vi "finlfinal1`.vi"() -> ()   [LabVIEW 2020]
uses:
  <vilib>/DAQmx/read.llb/DAQmx Read (Digital Bool 1Line 1Point).vi
  <vilib>/DAQmx/read.llb/DAQmx Read (Analog DBL 1Chan 1Samp).vi
  <vilib>/DAQmx/create/channels.llb/DAQmx Create Channel (AI-Voltage-Basic).vi
  <vilib>/DAQmx/create/channels.llb/DAQmx Create Channel (DI-Digital Input).vi
  <vilib>/Instr/_visa.llb/VISA Configure Serial Port (Instr).vi
  <vilib>/DAQmx/miscellaneous.llb/DAQmx Fill In Error Info.vi
  <vilib>/httpClient/PUTBuffer.vi
  <vilib>/httpClient/LabVIEWHTTPClient.lvlib
panel:
  in  "VISA resource name":refnum<visa-resource-name>
  in  "Bottle Presence":tag
  in  "Temperature":tag
  out "Temperature":dbl
  out "Humidity":dbl
  out "Temperature":dbl(knob) caption="Meter" scale=0.0..150.0
  out "Humidity Chart":dbl(graph)
  in  "Dispense Trigger":bool
  in  "Dispensing":bool
  out "error out":errorcluster
  out "Ready to Dispense":bool
  out "Temp Safe":bool
  out "Bottle Present":bool
  in  "stop":bool
  # "DOSEBOT"
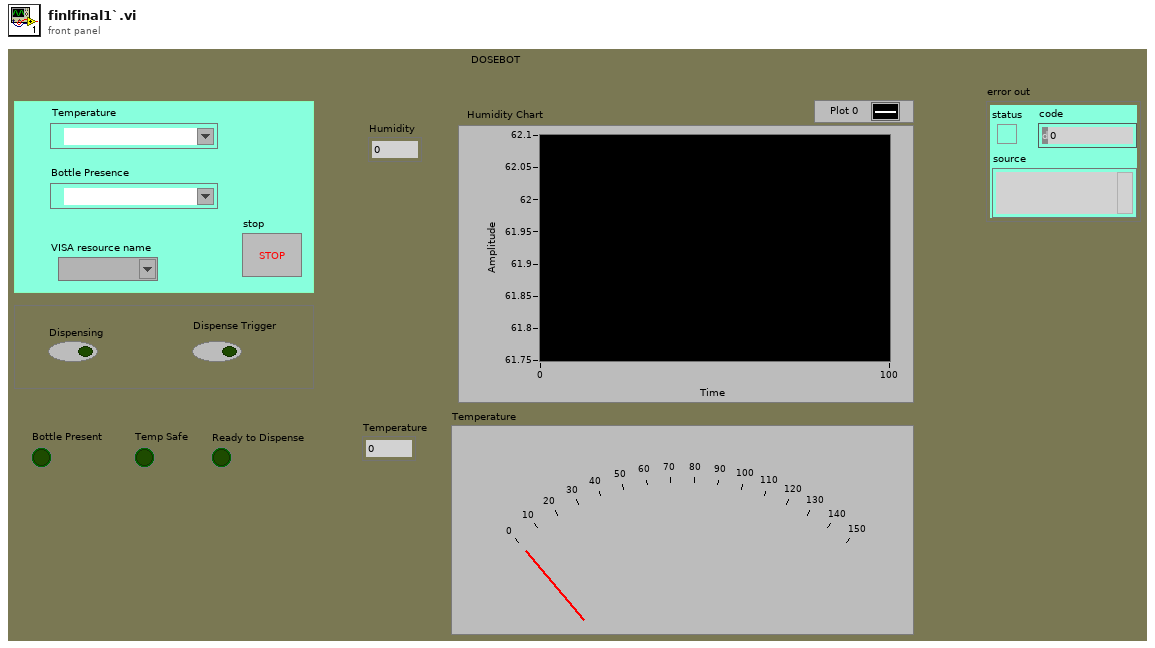
[diagram p1: front panel]
types:
  T1 = typedef "LabVIEWHTTPClient.lvlib/ClientHandle.ctl" = refnum<k1>
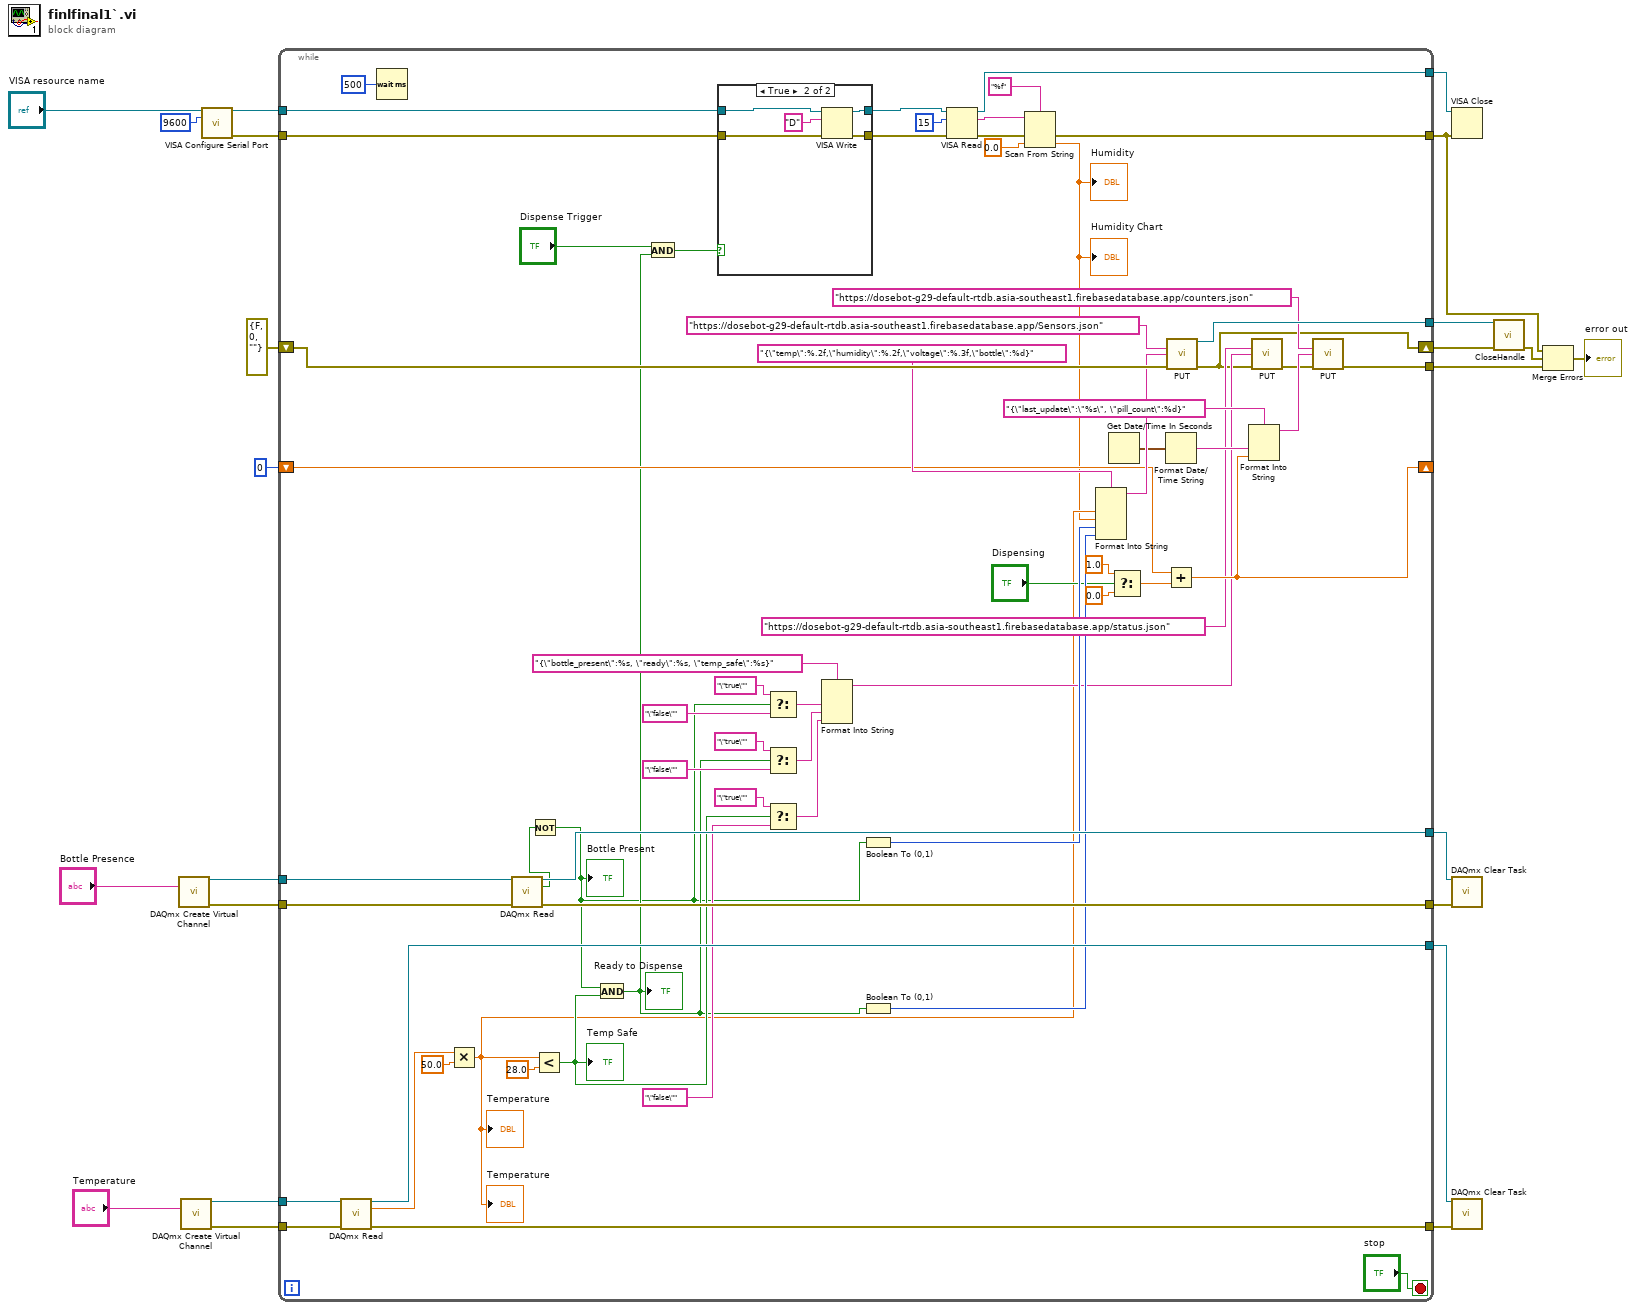
[diagram p0: block diagram]
diagram:
  n1 = call-poly <vilib>:"DAQmx Create Virtual Channel.vi"("lines"="Bottle Presence") -> ("task out"=w14:refnum<k21>, "error out"=w13:errorcluster)  [unwired: 13 in]
  n2 = call-poly <vilib>:"DAQmx Create Virtual Channel.vi"("physical channels"="Temperature") -> ("task out"=w19:refnum<k21>, "error out"=w18:errorcluster)  [unwired: 13 in]
  n3 = call-poly "VISA Configure Serial Port"("VISA resource name"="VISA resource name", "baud rate (9600)"=u32 9600) -> ("VISA resource name out"=w8:refnum<visa-resource-name>, "error out"=w7:errorcluster)  [unwired: 12 in]
  n4 = while {
    shift-right: [w38] -> w23
    shift-left: errorcluster {"status"=FALSE, "code"=0, "source"=""} ("error out") -> [w83]
    tunnel: [w84] -> w22
    tunnel: w19 -> [w82]
    tunnel: w18 -> [w81]
    tunnel: [w80] -> w17
    tunnel: [w79] -> w16
    tunnel: w14 -> [w78]
    tunnel: w13 -> [w77]
    tunnel: [w76] -> w12
    tunnel: [w75] -> w11
    tunnel: w8 -> [w31]
    tunnel: w7 -> [w30]
    tunnel: [w63] -> w5
    tunnel: [w68] -> w6
    shift-right: [w46] -> _
    shift-left: 0 -> [w48]
    tunnel: [w36] -> w1
    stop <- "stop" stop-if-true
    n5 = call-poly <vilib>:"DAQmx Read.vi"("task/channels in"=w82, "error in"=w81) -> ("task out"=w80:refnum<k21>, "data"=w73:dbl, "error out"=w79:errorcluster)  [unwired: 11 in]
    n6 = Wait (ms)(milliseconds to wait=u32 500) -> ()  [unwired: 1 out]
    n7 = Multiply(x=w73, y=50.0) -> (x*y=w27:dbl)
    "Temperature" <- w27
    "Temperature" <- w27
    n8 = call-poly <vilib>:"DAQmx Read.vi"("task/channels in"=w78, "error in"=w77) -> ("task out"=w76:refnum<k21>, "data"=w25:bool, "error out"=w75:errorcluster)  [unwired: 11 in]
    n9 = Not(x=w25) -> (.not. x?=w24:bool)
    "Bottle Present" <- w24
    n10 = Less?(x=w27, y=28.0) -> (x < y?=w55:bool)
    "Temp Safe" <- w55
    n11 = And(x=w24, y=w55) -> (x .and. y?=w34:bool)
    "Ready to Dispense" <- w34
    n12 = And(x="Dispense Trigger", y=w34) -> (x .and. y?=w33:bool)
    n13 = case shown="True" w33 {
      tunnel: w31 -> [w90 w94]
      tunnel: [w90 w93] -> w29
      tunnel: w30 -> [w89 w92]
      tunnel: [w89 w91] -> w28
      frame False {
      }
      frame True {
        n14 = VISA Write(VISA resource name=w94, write buffer="D", error in (no error)=w92) -> (VISA resource name out=w93:refnum<visa-resource-name>, error out=w91:errorcluster)  [unwired: 1 out]
      }
    }
    n15 = Select(t="\"true\"", s=w24, f="\"false\"") -> (s? t:f=w61:string)
    n16 = Select(t="\"true\"", s=w34, f="\"false\"") -> (s? t:f=w56:string)
    n17 = Select(t="\"true\"", s=w55, f="\"false\"") -> (s? t:f=w52:string)
    n18 = Format Into String(format string="{\"bottle_present\":%s, \"ready\":%s, \"temp_safe\":%s}", w61, w56, w52) -> (resulting string=w40:string)  [unwired: 2 in, 1 out]
    n19 = Boolean To (0,1)(Boolean=w24) -> (0, 1=w69:i16)
    n20 = Boolean To (0,1)(Boolean=w34) -> (0, 1=w70:i16)
    n21 = VISA Read(VISA resource name=w29, byte count=u32 15, error in (no error)=w28) -> (VISA resource name out=w68:refnum<visa-resource-name>, read buffer=w32:string, error out=w64:errorcluster)  [unwired: 1 out]
    n22 = Scan From String(format string="%f", input string=w32, error in=w64, default 1=0.0 ("default (0 dbl)")) -> (error out=w63:errorcluster, output 1=w26:dbl)  [unwired: 1 in, 2 out]
    "Humidity Chart" <- w26
    "Humidity" <- w26
    n23 = Format Into String(format string="{\"temp\":%.2f,\"humidity\":%.2f,\"voltage\":%.3f,\"bottle\":%d}", w27, w26, w69, w70) -> (resulting string=w71:string)  [unwired: 2 in, 1 out]
    n24 = Get Date/Time In Seconds() -> (seconds since 1Jan1904=w49:timestamp)
    n25 = Select(t=1.0, s="Dispensing", f=0.0) -> (s? t:f=w47:dbl)
    n26 = Format Date/Time String(seconds (now)=w49) -> (date/time string=w50:string)  [unwired: 2 in]
    n27 = Add(x=w48, y=w47) -> (x+y=w46:dbl)
    n28 = call-poly <vilib>:"PUT.vi"("url"="https://dosebot-g29-default-rtdb.asia-southeast1.firebasedatabase.app/Sensors.json", "buffer"=w71, "error in (no error)"=w83) -> ("client handle out"=w84:T1, "error out"=w38:errorcluster)  [unwired: 9 in, 2 out]
    n29 = Format Into String(format string="{\"last_update\":\"%s\", \"pill_count\":%d}", w50, w46) -> (resulting string=w39:string)  [unwired: 2 in, 1 out]
    n30 = call-poly <vilib>:"PUT.vi"("url"="https://dosebot-g29-default-rtdb.asia-southeast1.firebasedatabase.app/status.json", "buffer"=w40, "error in (no error)"=w38) -> ("error out"=w37:errorcluster)  [unwired: 9 in, 3 out]
    n31 = call-poly <vilib>:"PUT.vi"("url"="https://dosebot-g29-default-rtdb.asia-southeast1.firebasedatabase.app/counters.json", "buffer"=w39, "error in (no error)"=w37) -> ("error out"=w36:errorcluster)  [unwired: 9 in, 3 out]
  }
  n32 = VISA Close(VISA resource name=w6, error in (no error)=w5) -> ()  [unwired: 1 out]
  n33 = call <vilib>:"DAQmx Clear Task.vi"("task in"=w12, "error in"=w11) -> ()  [unwired: 13 in, 1 out]
  n34 = call <vilib>:"DAQmx Clear Task.vi"("task in"=w17, "error in"=w16) -> ()  [unwired: 13 in, 1 out]
  n35 = call <vilib>:"CloseHandle.vi"("client handle"=w22, "error in (no error)"=w23) -> ("error out"=w4:errorcluster)  [unwired: 13 in]
  n36 = Merge Errors(w5, w4, w1) -> (→"error out":errorcluster)
